vi "Custom Assertion Failure Message.vi"() -> ()   [LabVIEW 2017, in "Assertion.Tests.lvlib" / "Assert Not Equals.lvlib"]
uses:
  Assert Not Equals.lvlib
  4c0fa4f8-e8bf-466f-afde-48ab27d81456.vi
  Constraint/IsEqual/IsEqual.lvclass
  C:/Users/de200256/Code/logmanoriginal/lvunit/Constraint/Constraint/Constraint.lvclass
  Constraint/IsEqual/Create.vi
  Constraint/LogicalNot/LogicalNot.lvclass
  Constraint/UnaryOperator/UnaryOperator.lvclass
  Assertion/Assertion.lvlib
panel:
  out "error out":errorcluster
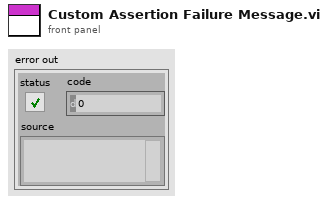
[diagram p1: front panel]
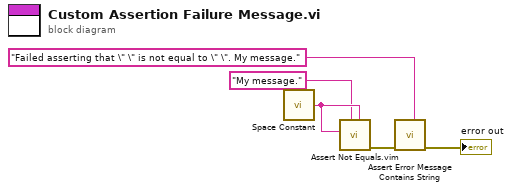
[diagram p0: block diagram]
diagram:
  n1 = call <vilib>:"Space Constant.vi"() -> ("String"=w2:string)
  n2 = call "Assert Not Equals.vim"("Expected"=w2, "Message (\"\")"="My message.", "Actual"=w2) -> ("error out"=w5:errorcluster)  [unwired: 8 in]
  n3 = call "Assert Error Message Contains String.vi"("Expected"="Failed asserting that \" \" is not equal to \" \". My message." ("y"), "error in (no error)"=w5) -> ("error out"=→"error out":errorcluster)  [unwired: 9 in]
